vi "Configure.vi"(8 "error in (no error)":errorcluster, 11 "GRMActor in":refnum<class "DataLoggerUI.lvclass">) -> (0 "error out":errorcluster, 3 "GRMActor out":refnum<class "DataLoggerUI.lvclass">)   [LabVIEW 2020, in "DataLoggerUI.lvlib" / "DataLoggerUI.lvclass"]
uses:
  DataLoggerUI.lvclass
  DataLoggerUI.lvclass/DataLoggerUI.ctl
  Hardware Abstraction Layer/Component/GenericActor/GenericActor/GenericController.lvclass
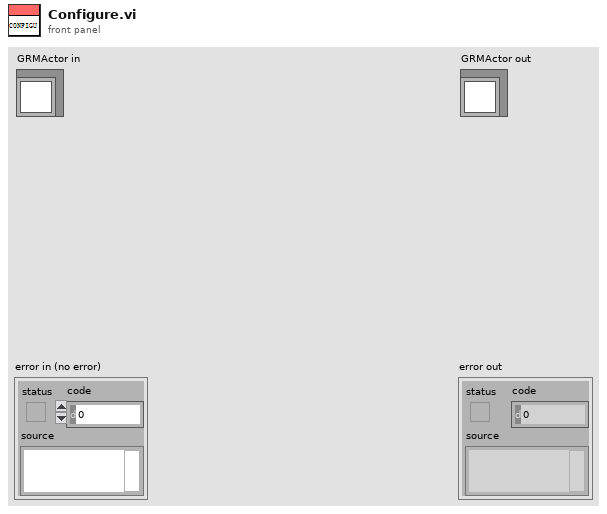
[diagram p1: front panel]
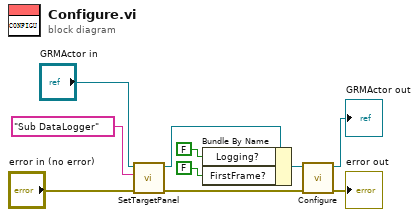
[diagram p0: block diagram]
diagram:
  n1 = call-dynamic "SetTargetPanel.vi"("error in (no error)"="error in (no error)", "TargetPanel"="Sub DataLogger" ("Panel"), "GRMActor in"="GRMActor in") -> ("error out"=w3:errorcluster, "GRMActor out"=w8:refnum<class "DataLoggerUI.lvclass">)  [unwired: 7 in]
  n2 = Bundle By Name(cluster=w8, "Logging?"=FALSE, "FirstFrame?"=FALSE) -> (w4:refnum<class "DataLoggerUI.lvclass">)
  n3 = call-parent "Configure.vi"("error in (no error)"=w3, "GRMActor in"=w4) -> ("error out"=→"error out":errorcluster, "GRMActor out"=→"GRMActor out":refnum<class "DataLoggerUI.lvclass">)  [unwired: 8 in]
